vi "CheckIfLensThicknessInRange.vi"(9 "Thickness range":dbl, 10 "Wanted thickness":dbl, 11 "Lens thickness":dbl) -> (3 "Lens thickness in range?":bool)   [LabVIEW 2013]
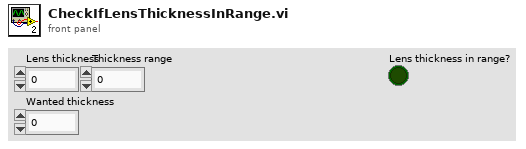
[diagram p1: front panel]
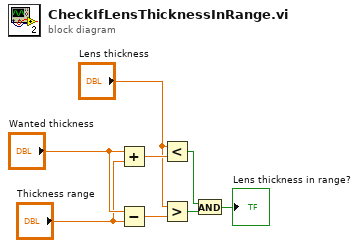
[diagram p0: block diagram]
diagram:
  n1 = Add(x="Wanted thickness", y="Thickness range") -> (x+y=w6:dbl)
  n2 = Subtract(x="Wanted thickness", y="Thickness range") -> (x-y=w5:dbl)
  n3 = Less?(x="Lens thickness", y=w6) -> (x < y?=w7:bool)
  n4 = Greater?(x="Lens thickness", y=w5) -> (0:w8:bool)
  n5 = And(x=w7, y=w8) -> (x .and. y?=→"Lens thickness in range?":bool)
